vi "Rendezvous Name & Ref DB.vi"(1 "Action":T1, 2 "Rendezvous Name":string, 3 "rendezvous ref in":T2) -> (0 "rendezvous  ref out":T2)   [LabVIEW 2010]
uses:
  Rendezvous Name & Ref DB Action.ctl
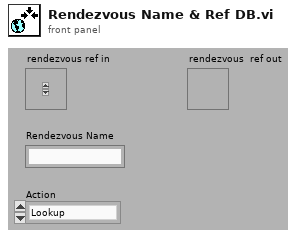
[diagram p1: front panel]
types:
  T1 = typedef "Rendezvous Name & Ref DB Action.ctl" = enum16{"Lookup", "Insert", "Remove"}
  T2 = typedef "Rendezvous RefNum" = refnum<k1>
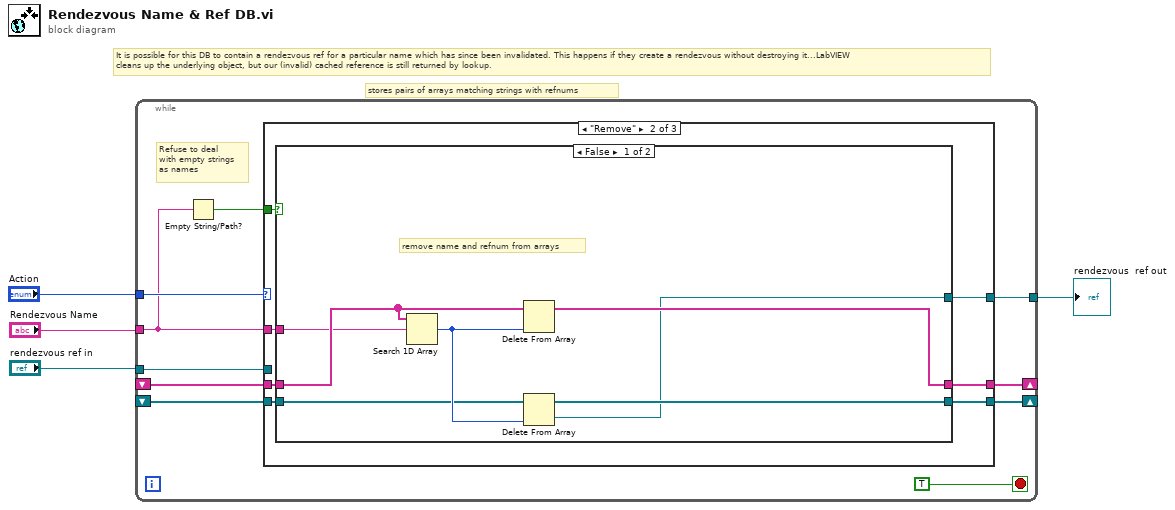
[diagram p0: block diagram]
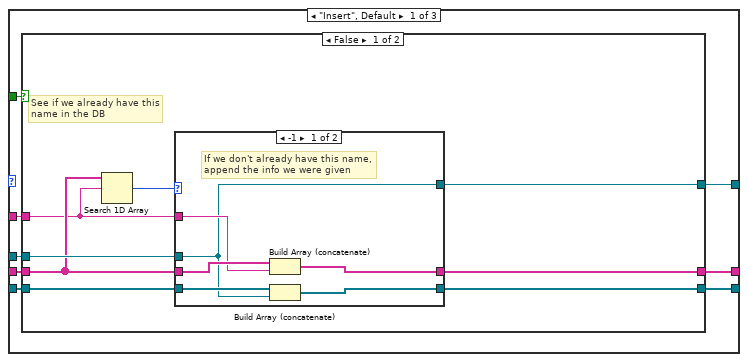
[diagram p2: hidden frame]
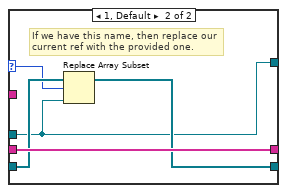
[diagram p3: hidden frame]
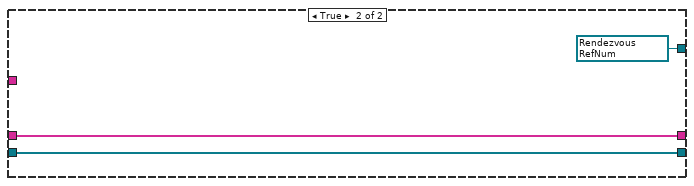
[diagram p5: hidden frame]
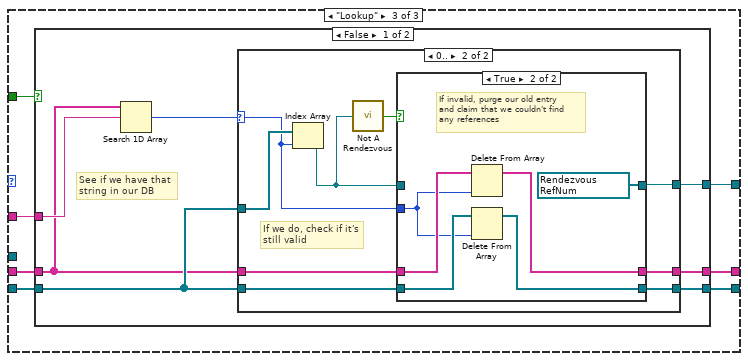
[diagram p6: hidden frame]
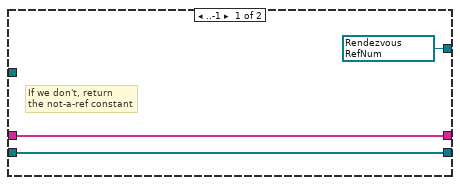
[diagram p7: hidden frame]
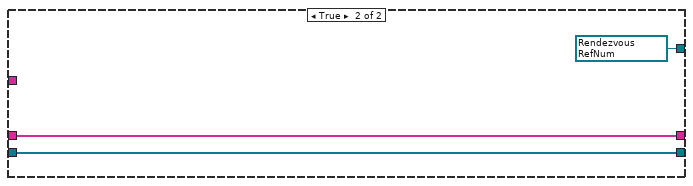
[diagram p9: hidden frame]
diagram:
  # "It is possible for this DB to contain a rendezvous ref for a particular name which has since been invalidated. This happens if they create a rendezvous without destroying it...LabVIEW\ncleans up the underlying object, but our (invalid) cached reference is still returned by lookup."
  # "stores pairs of arrays matching strings with refnums"
  n1 = while {
    shift-right: [w10] -> _
    shift-left: _ -> [w9]
    shift-right: [w12] -> _
    shift-left: _ -> [w11]
    tunnel: "Action" -> [w14]
    tunnel: "Rendezvous Name" -> [w5]
    tunnel: "rendezvous ref in" -> [w13]
    tunnel: [w7] -> w2
    stop <- TRUE stop-if-true
    # "Refuse to deal\nwith empty strings\nas names"
    n2 = Empty String/Path?(string/path=w5) -> (empty?=w6:bool)
    n3 = case shown="\"Remove\"" w14 {
      tunnel: w5 -> [w16 w46 w63]
      tunnel: w13 -> [w22 _ _]
      tunnel: [w21 w50 w65] -> w12
      tunnel: w11 -> [w20 w51 w66]
      tunnel: [w19 w48 w64] -> w10
      tunnel: w9 -> [w18 w49 w67]
      tunnel: [w17 w47 w68] -> w7
      tunnel: w6 -> [w15 w45 w62]
      frame "Insert", Default {
        n4 = case shown="False" w15 {
          tunnel: w22 -> [w30 w44]
          tunnel: [w29 w42] -> w21
          tunnel: w20 -> [w28 w42]
          tunnel: [w27 w43] -> w19
          tunnel: w18 -> [w26 w43]
          tunnel: w16 -> [w25 _]
          tunnel: [w23 w44] -> w17
          frame False {
            # "See if we already have this\nname in the DB"
            n5 = Search 1D Array(1D array=w26, element=w25) -> (index of element=w24:i32)  [unwired: 1 out]
            n6 = case shown="-1" w24 {
              selector: w24 -> [_ w39]
              tunnel: w30 -> [w32 w37]
              tunnel: [w36 w38] -> w29
              tunnel: w28 -> [w35 w40]
              tunnel: [w31 w41] -> w27
              tunnel: w26 -> [w34 w41]
              tunnel: w25 -> [w33 _]
              tunnel: [w32 w37] -> w23
              frame -1 {
                # "If we don't already have this name,\nappend the info we were given"
                n7 = Build Array (concatenate)(w34, w33) -> (w31:string[])
                n8 = Build Array (concatenate)(w35, w32) -> (w36:T2[])
              }
              frame 1, Default {
                # "If we have this name, then replace our \ncurrent ref with the provided one."
                n9 = Replace Array Subset(array=w40, new element=w37, index=w39) -> (w38:T2[])
              }
            }
          }
          frame True {
          }
        }
      }
      frame "Remove" {
        n10 = case shown="False" w45 {
          tunnel: w51 -> [w57 w61]
          tunnel: [w56 w61] -> w50
          tunnel: w49 -> [w55 w60]
          tunnel: [w54 w60] -> w48
          tunnel: [w53 w59] -> w47
          tunnel: w46 -> [w52 _]
          frame False {
            # "remove name and refnum from arrays"
            n11 = Search 1D Array(1D array=w55, element=w52) -> (index of element=w58:i32)  [unwired: 1 out]
            n12 = Delete From Array(array=w55, index=w58) -> (array with subset deleted=w54:string[])  [unwired: 1 in, 1 out]
            n13 = Delete From Array(array=w57, index=w58) -> (deleted portion=w53:T2, array with subset deleted=w56:T2[])  [unwired: 1 in]
          }
          frame True {
            w59 = T2 refnum items=["rendezvous"] ("rendezvous ref in")
          }
        }
      }
      frame "Lookup" {
        n14 = case shown="False" w62 {
          tunnel: [w75 w97] -> w68
          tunnel: w67 -> [w71 w99]
          tunnel: w63 -> [w74 _]
          tunnel: w66 -> [w72 w98]
          tunnel: [w73 w98] -> w65
          tunnel: [w70 w99] -> w64
          frame False {
            # "See if we have that \nstring in our DB"
            n15 = Search 1D Array(1D array=w71, element=w74) -> (index of element=w69:i32)  [unwired: 1 out]
            n16 = case shown="0.." w69 {
              selector: w69 -> [_ w79]
              tunnel: [w76 w86] -> w75
              tunnel: w72 -> [_ w87]
              tunnel: [w77 w82] -> w73
              tunnel: w72 -> [w77 w85]
              tunnel: w71 -> [w78 w84]
              tunnel: [w78 w83] -> w70
              frame ..-1 {
                w76 = T2 refnum items=["rendezvous"] ("rendezvous ref in")
                # "If we don't, return\nthe not-a-ref constant"
              }
              frame 0.. {
                # "If we do, check if it's\nstill valid"
                n17 = Index Array(array=w87, index=w79) -> (element=w81:T2)
                n18 = call "Not A Rendezvous.vi"("rendezvous"=w81) -> ("not a rendezvous"=w80:bool)
                n19 = case shown="True" w80 {
                  tunnel: [w90 w91] -> w86
                  tunnel: w81 -> [w90 _]
                  tunnel: w79 -> [_ w92]
                  tunnel: w85 -> [w88 w95]
                  tunnel: w84 -> [w89 w96]
                  tunnel: [w89 w93] -> w83
                  tunnel: [w88 w94] -> w82
                  frame False {
                    # "If it is valid, pass it through"
                  }
                  frame True {
                    w91 = T2 refnum items=["rendezvous"] ("rendezvous ref in")
                    # "If invalid, purge our old entry\nand claim that we couldn't find\nany references"
                    n20 = Delete From Array(array=w96, index=w92) -> (array with subset deleted=w93:string[])  [unwired: 1 in, 1 out]
                    n21 = Delete From Array(array=w95, index=w92) -> (array with subset deleted=w94:T2[])  [unwired: 1 in, 1 out]
                  }
                }
              }
            }
          }
          frame True {
            w97 = T2 refnum items=["rendezvous"] ("rendezvous ref in")
          }
        }
      }
    }
  }
  "rendezvous  ref out" <- w2
